vi "19.8-Morphological .vi"() -> ()   [LabVIEW 2020]
doc: "Uses the Median Filter VI to analyze pulses in the presence of noise. The example generates a pulse contaminated with Gaussian noise and applies a median filter. For comparison purposes, the VI computes the pulse parameters of the filtered pulse."
uses:
  <vilib>/Analysis/NI_AALPro.lvlib
  <vilib>/Analysis/NI_AALBase.lvlib
  <vilib>/Analysis/NI_AAL_Filter.lvlib
panel:
  in  "Structure Element":dbl[](array[numeric])=[0.0, 0.0, 0.0, 0.0, 0.0, 0.0, 0.0, 0.0, 0.0, 0.0]
  in  "Stop":bool
  out "Amplitude (est)":dbl format="%#.2g"
  in  "Amplitude":dbl=5.0 format="%#.6g"
  out "Delay (est)":dbl format="%#.2g"
  in  "Delay (samples)":i32=64
  out "Width (est)":dbl format="%#.2g"
  in  "Width (samples)":i32=32
  out "Graph":dbl[][](graph)
  in  "Samples":i32=128
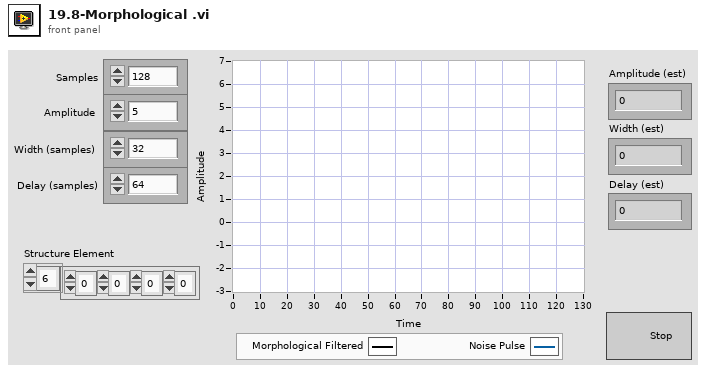
[diagram p1: front panel]
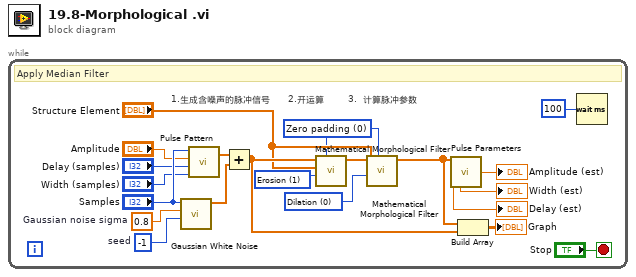
[diagram p0: block diagram]
diagram:
  n1 = while {
    stop <- "Stop" stop-if-true
    w3 = u16 0 items=["Dilation", "Erosion"] ("operation type")
    w6 = u16 1 items=["Dilation", "Erosion"] ("operation type")
    w1 = u16 0 items=["Zero padding", "Symmetric", "Periodic"] ("X extension type")
    w21 = 0.8  # Gaussian noise sigma
    w8 = -1  # seed
    # "1.生成含噪声的脉冲信号      2.开运算        3.  计算脉冲参数"
    # "Apply Median Filter"
    n2 = call <vilib>:"Gaussian White Noise.vi"("seed"=w8, "standard deviation"=w21, "samples"="Samples") -> ("Gaussian noise pattern"=w20:dbl[])  [unwired: 7 in, 1 out]
    n3 = call <vilib>:"Pulse Pattern.vi"("width"="Width (samples)", "delay"="Delay (samples)", "amplitude"="Amplitude", "samples"="Samples") -> ("Pulse Pattern"=w13:dbl[])  [unwired: 1 out]
    n4 = Add(x=w13, y=w20) -> (x+y=w7:dbl[])
    n5 = call <vilib>:"Mathematical Morphological Filter.vi"("X extension type"=w1, "operation type"=w6, "Structure Element"="Structure Element", "X"=w7) -> ("Filtered X"=w5:dbl[])  [unwired: 6 in, 1 out]
    n6 = call <vilib>:"Mathematical Morphological Filter.vi"("X extension type"=w1, "operation type"=w3, "Structure Element"="Structure Element", "X"=w5) -> ("Filtered X"=w4:dbl[])  [unwired: 6 in, 1 out]
    n7 = call <vilib>:"Pulse Parameters.vi"("X"=w4) -> ("amplitude"=→"Amplitude (est)":dbl, "delay"=→"Delay (est)":dbl, "duration"=→"Width (est)":dbl)  [unwired: 4 in, 8 out]
    n8 = Build Array(w4, w7) -> (→"Graph":dbl[][])
    n9 = Wait (ms)(milliseconds to wait=u32 100) -> ()  [unwired: 1 out]
  }
